vi "Set_Reset_DB0_11.vi"(2 "error in":errorcluster, 3 "device name":tag="Dev0", 4 "DB0-11":u16) -> (0 "error out":errorcluster)   [LabVIEW 2017]
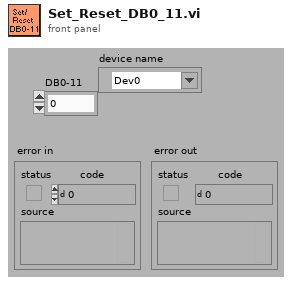
[diagram p1: front panel]
types:
  T1 = enum16{"Reset", "Update U1", "Update U2", "Update U3", "Read all", "Update U1&U2"}
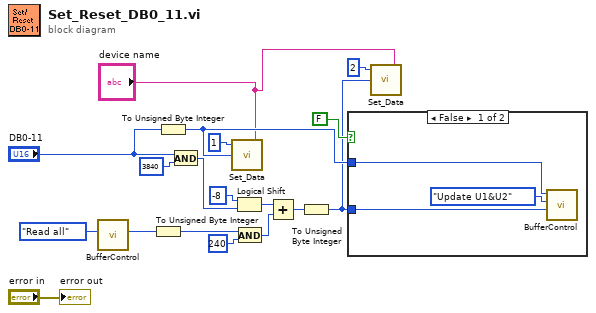
[diagram p0: block diagram]
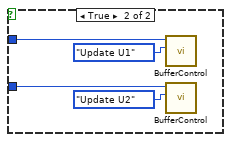
[diagram p2: hidden frame]
diagram:
  n1 = call "BufferControl.vi"("Enum"=T1."Read all") -> ("U2BuffRead"=w13:u8)  [unwired: 3 in, 3 out]
  n2 = To Unsigned Byte Integer(number=w13) -> (unsigned 8bit integer=w12:u8)
  n3 = To Unsigned Byte Integer(number="DB0-11") -> (unsigned 8bit integer=w3:u8)
  n4 = And(x="DB0-11", y=u16 3840) -> (x .and. y?=w8:u16)
  n5 = call "Set_Data.vi"("device name"="device name", "Data"=w3, "Ch"=u8 1) -> ()  [unwired: 1 in, 1 out]
  n6 = Logical Shift(y=i16 -8, x=w8) -> (x << y=w9:u16)
  n7 = And(x=w12, y=u16 240) -> (x .and. y?=w11:u16)
  n8 = Add(x=w9, y=w11) -> (x+y=w6:u16)
  n9 = To Unsigned Byte Integer(number=w6) -> (unsigned 8bit integer=w2:u8)
  n10 = case shown="False" FALSE ("Case Constant\n(See Context Help)") {
    tunnel: w3 -> [w20 w25]
    tunnel: w2 -> [w19 w24]
    frame False {
      n11 = call "BufferControl.vi"("Data 2"=w19, "Enum"=T1."Update U1&U2", "Data"=w20) -> ()  [unwired: 1 in, 4 out]
    }
    frame True {
      n12 = call "BufferControl.vi"("Enum"=T1."Update U1", "Data"=w25) -> ()  [unwired: 2 in, 4 out]
      n13 = call "BufferControl.vi"("Enum"=T1."Update U2", "Data"=w24) -> ()  [unwired: 2 in, 4 out]
    }
  }
  n14 = call "Set_Data.vi"("device name"="device name", "Data"=w2, "Ch"=u8 2) -> ()  [unwired: 1 in, 1 out]
  "error out" <- "error in"
